vi "Enqueue Message.vi"(6 "priority nessage":bool, 8 "error in":errorcluster, 9 "message data":variant, 10 "message":string, 11 "message queue":refnum<queue>) -> (0 "error out":errorcluster, 3 "dup message queue":refnum<queue>)   [LabVIEW 2024, in "DSA_CFG_ACQ.lvlib" / "SFPMessage Queue.lvlib"]
doc: "For a regular message, enqueue the message. For a priority message, enqueue it at the front of the queue."
uses:
  SFPMessage Queue.lvlib
  Message Cluster.ctl
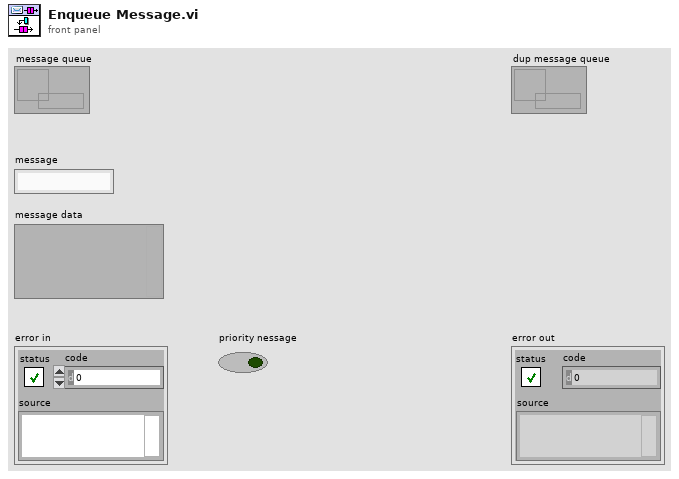
[diagram p1: front panel]
types:
  T1 = typedef "DSA_CFG_ACQ.lvlib/SFPMessage Queue.lvlib/Message Cluster.ctl" = cluster{"Message":string, "Message Data":variant}
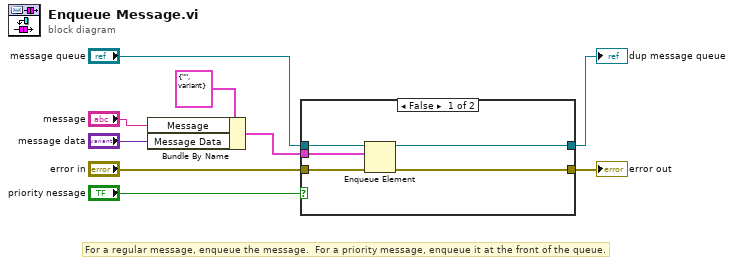
[diagram p0: block diagram]
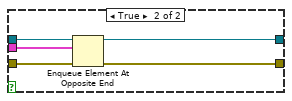
[diagram p2: hidden frame]
diagram:
  # "For a regular message, enqueue the message.  For a priority message, enqueue it at the front of the queue."
  n1 = Bundle By Name(cluster=T1 {"Message"="", "Message Data"=variant} ("Message Cluster"), "Message"="message", "Message Data"="message data") -> (w3:T1)
  n2 = case shown="False" "priority nessage" {
    tunnel: "error in" -> [w14 w19]
    tunnel: [w13 w18] -> w4
    tunnel: "message queue" -> [w12 w17]
    tunnel: w3 -> [w11 w16]
    tunnel: [w10 w15] -> w1
    frame False {
      n3 = Enqueue Element(queue=w12, element=w11, error in (no error)=w14) -> (queue out=w10:refnum<queue>, error out=w13:errorcluster)  [unwired: 1 in, 1 out]
    }
    frame True {
      n4 = Enqueue Element At Opposite End(queue=w17, element=w16, error in (no error)=w19) -> (queue out=w15:refnum<queue>, error out=w18:errorcluster)  [unwired: 1 in, 1 out]
    }
  }
  "error out" <- w4
  "dup message queue" <- w1
